vi "iWorx Thermistor Scaling.vi"(4 "Rseries (10k)":dbl=10000.0, 5 "Calibration Coefficients":cluster{"Ka":dbl, "Kb":dbl, "Kc":dbl}[](array[cluster])=[{"Ka"=0.00073998, "Kb"=0.00027874, "Kc"=9.2632e-08}, {"Ka"=0.00073998, "Kb"=0.00027874, "Kc"=9.2632e-08}] {"Ka" format="%#.4e"}, 6 "Set Point Temp":dbl=5.0, 7 "Set":bool, 8 "Clear":bool, 9 "Vref(10)":dbl=10.0, 10 "Vt Measured":dbl[](array[numeric])=[0.0, 0.0, 0.0, 0.0, 0.0, 0.0, 0.0, 0.0, 0.0], 11 "Use One K Set (t)":bool=TRUE) -> (1 "Offsets":dbl[](array[numeric]), 2 "Temps":dbl[](array[numeric]))   [LabVIEW 2012]
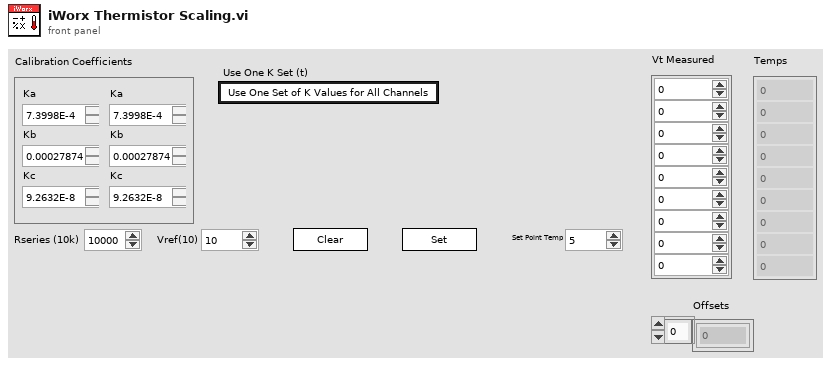
[diagram p1: front panel]
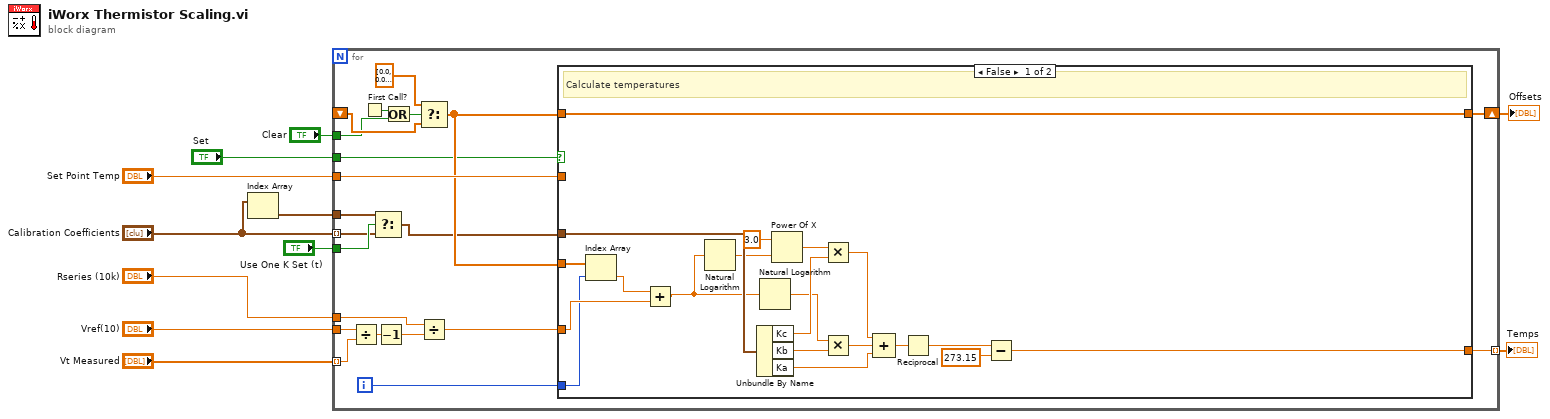
[diagram p0: block diagram]
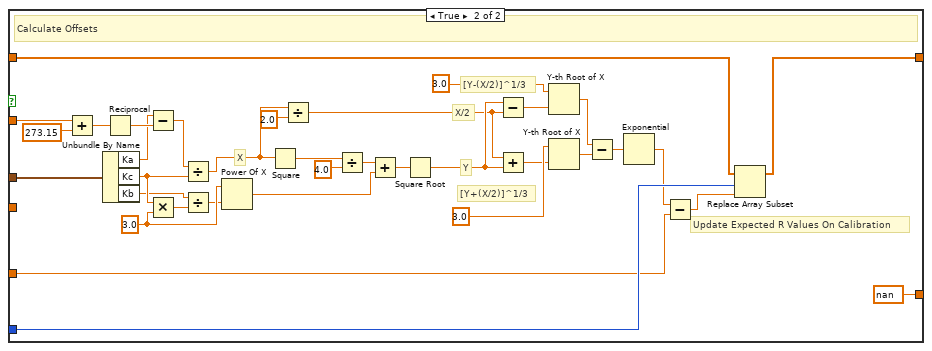
[diagram p2: hidden frame]
diagram:
  n1 = Index Array(array="Calibration Coefficients") -> (element=w1:cluster{"Ka":dbl, "Kb":dbl, "Kc":dbl})  [unwired: 1 in]
  n2 = for {
    tunnel: "Set Point Temp" -> [w32]
    tunnel: "Vt Measured" -> [w31] mode=indexing
    tunnel: "Vref(10)" -> [w30]
    tunnel: "Rseries (10k)" -> [w27]
    tunnel: [w26] -> w9 mode=indexing
    shift-right: [w25] -> w6
    shift-left: _ -> [w24]
    tunnel: "Set" -> [w19]
    tunnel: "Clear" -> [w18]
    tunnel: "Use One K Set (t)" -> [w15]
    tunnel: "Calibration Coefficients" -> [w14] mode=indexing
    tunnel: w1 -> [w13]
    i -> [w22]
    n3 = Divide(x=w30, y=w31) -> (x/y=w29:dbl)
    n4 = First Call?() -> (First Call?: T/F=w17:bool)
    n5 = Select(t=w13, s=w15, f=w14) -> (s? t:f=w12:cluster{"Ka":dbl, "Kb":dbl, "Kc":dbl})
    n6 = Decrement(x=w29) -> (x-1=w28:dbl)
    n7 = Or(x=w17, y=w18) -> (x .or. y?=w16:bool)
    n8 = Select(t=dbl[] [0.0, 0.0, 0.0, 0.0, 0.0, 0.0, 0.0] ("Ref, Vt Measured 2"), s=w16, f=w24) -> (s? t:f=w20:dbl[])
    n9 = Divide(x=w27, y=w28) -> (x/y=w21:dbl)
    n10 = case shown="False" w19 {
      tunnel: w32 -> [_ w87]
      tunnel: w12 -> [w43 w60]
      tunnel: [w39 nan] -> w26
      tunnel: w20 -> [w38 w58]
      tunnel: w22 -> [w34 w57]
      tunnel: [w38 w56] -> w25
      tunnel: w21 -> [w36 w53]
      tunnel: w20 -> [w35 _]
      frame False {
        # "Calculate temperatures"
        n11 = Index Array(array=w35, index=w34) -> (element=w33:dbl)
        n12 = Add(x=w33, y=w36) -> (x+y=w37:dbl)
        n13 = Natural Logarithm(1:w37) -> (0:w42:dbl)
        n14 = Unbundle By Name(w43) -> ("Kc"=w52:dbl, "Kb"=w51:dbl, "Ka"=w50:dbl)
        n15 = Natural Logarithm(1:w37) -> (0:w45:dbl)
        n16 = Power Of X(1:w42, 2:3.0 ("y")) -> (0:w40:dbl)
        n17 = Multiply(x=w40, y=w52) -> (x*y=w46:dbl)
        n18 = Multiply(x=w45, y=w51) -> (x*y=w47:dbl)
        n19 = Compound Arithmetic op=ADD(w46, w47, w50) -> (w48:dbl)
        n20 = Reciprocal(x=w48) -> (1/x=w49:dbl)
        n21 = Subtract(x=w49, y=273.15) -> (x-y=w39:dbl)
      }
      frame True {
        w81 = 3.0 ("x")
        # "Update Expected R Values On Calibration"
        # "[Y+(X/2)]^1/3"
        # "[Y-(X/2)]^1/3"
        # "X/2"
        # "Y"
        # "X"
        # "Calculate Offsets"
        n22 = Add(x=w87, y=273.15) -> (x+y=w79:dbl)
        n23 = Unbundle By Name(w60) -> ("Ka"=w76:dbl, "Kc"=w75:dbl, "Kb"=w73:dbl)
        n24 = Reciprocal(x=w79) -> (1/x=w78:dbl)
        n25 = Subtract(x=w76, y=w78) -> (x-y=w77:dbl)
        n26 = Multiply(x=w75, y=w81) -> (x*y=w74:dbl)
        n27 = Divide(x=w77, y=w75) -> (x/y=w68:dbl)
        n28 = Divide(x=w73, y=w74) -> (x/y=w80:dbl)
        n29 = Power Of X(1:w80, 2:w81) -> (0:w82:dbl)
        n30 = Square(x=w68) -> (x^2=w69:dbl)
        n31 = Divide(x=w68, y=2.0) -> (x/y=w65:dbl)
        n32 = Divide(x=w69, y=4.0) -> (x/y=w71:dbl)
        n33 = Add(x=w71, y=w82) -> (x+y=w70:dbl)
        n34 = Square Root(x=w70) -> (sqrt(x)=w66:dbl)
        n35 = Subtract(x=w66, y=w65) -> (x-y=w83:dbl)
        n36 = Add(x=w65, y=w66) -> (x+y=w85:dbl)
        n37 = Y-th Root of X(1:w83, 2:3.0 ("x")) -> (0:w64:dbl)
        n38 = Y-th Root of X(1:w85, 2:3.0 ("x")) -> (0:w63:dbl)
        n39 = Subtract(x=w64, y=w63) -> (x-y=w62:dbl)
        n40 = Exponential(1:w62) -> (0:w55:dbl)
        n41 = Subtract(x=w55, y=w53) -> (x-y=w54:dbl)
        n42 = Replace Array Subset(array=w58, new element=w54, index=w57) -> (w56:dbl[])
      }
    }
  }
  "Temps" <- w9
  "Offsets" <- w6
